vi "PH_PowerUnit_BaseClass.write PSDB.vi"(0 "i ref in":refnum<vi>, 5 "error IO":errorcluster) -> (14 "i ref out":refnum<vi>, 19 "error out":errorcluster)   [LabVIEW 2014, in "PH_PowerUnit_BaseClass.lvlib"]
doc: "This is the proc case which writes data to the PHELIX shot data base."
uses:
  PH_PowerUnit_BaseClass.lvlib
  PH_PSDBWriter/PH_PSDBWriter.lvlib
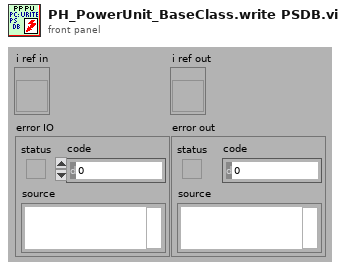
[diagram p1: front panel]
types:
  T1 = typedef "PH_PSDBWriter.lvlib/PH_PSDBWriter.Boolean dataset.ctl" = cluster{"name":string, "data":bool, "unit":string}
  T2 = typedef "PH_PSDBWriter.lvlib/PH_PSDBWriter.String dataset.ctl" = cluster{"name":string, "data":string, "unit":string}
  T3 = typedef "PH_PSDBWriter.lvlib/PH_PSDBWriter.PSDB Dataset.ctl" = cluster{"Version":i32, "2D data Input":T4[], "Boolean Input":T1[], "Image Input":T6[], "Numeric Input":T8[], "String Input":T2[]}
  T4 = typedef "PH_PSDBWriter.lvlib/PH_PSDBWriter.2D dataset.ctl" = cluster{"name":string, "data":dbl[][], "axis description":T5}
  T5 = typedef "PSDB.lvlib/PSDB_AxisDescription.ctl" = cluster{"x axis label":string, "y axis label":string, "x axis unit":string, "y axis unit":string}
  T6 = typedef "PH_PSDBWriter.lvlib/PH_PSDBWriter.Image dataset.ctl" = cluster{"name":string, "data":T7, "unit":string}
  T7 = typedef "IMAQ Image.ctl" = refnum<image>
  T8 = typedef "PH_PSDBWriter.lvlib/PH_PSDBWriter.Numeric dataset.ctl" = cluster{"name":string, "data":dbl, "unit":string}
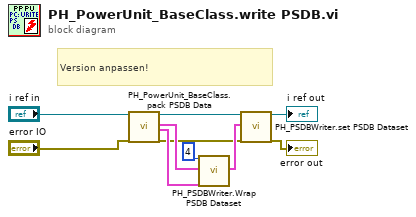
[diagram p0: block diagram]
diagram:
  # "Version anpassen!"
  n1 = call "PH_PowerUnit_BaseClass.pack PSDB Data.vi"("VI in"="i ref in", "error in (no error)"="error IO") -> ("VI out"=w2:refnum<vi>, "PSDB Boolean Data Array"=w5:T1[], "PSDB String Data Array"=w4:T2[], "error out"=w1:errorcluster)  [unwired: 14 in]
  n2 = call "PH_PSDBWriter.Wrap PSDB Dataset.vi"("Version"=4, "Boolean Input"=w5, "String Input"=w4) -> ("PSDB Dataset"=w3:T3)  [unwired: 16 in]
  n3 = call "PH_PSDBWriter.set PSDB Dataset.vi"("VI in"=w2, "PSDB Dataset"=w3, "error in (no error)"=w1) -> ("VI out"=→"i ref out":refnum<vi>, "error out"=→"error out":errorcluster)  [unwired: 15 in]
